vi "LaserReadContinuous.vi"() -> ()   [LabVIEW 2018]
uses:
  <vilib>/myRIO/Instrument Drivers/Onboard IO/I2C/typedefs/I2C User Configuration.ctl
  <vilib>/myRIO/Instrument Drivers/Onboard IO/I2C/typedefs/I2C Transfer Rate.ctl
  <vilib>/myRIO/Instrument Drivers/Onboard IO/I2C/typedefs/I2C Reference.ctl
  <vilib>/myRIO/Common/Instrument Driver Framework/Utilities/typedefs/myRIO Generic Hardware Reference.ctl
  <vilib>/myRIO/Common/Instrument Driver Framework/Utilities/typedefs/Hardware Version Enum.ctl
  <vilib>/myRIO/Common/Instrument Driver Framework/Utilities/typedefs/myRIO v1.0 Reference.ctl
  <vilib>/myRIO/Common/Instrument Driver Framework/Utilities/typedefs/Generic FPGA Reference.ctl
  <vilib>/myRIO/Common/Instrument Driver Framework/myRIO v1.0/I2C/typedefs/I2C Channels Enum.ctl
  <vilib>/myRIO/Instrument Drivers/Onboard IO/I2C/typedefs/I2C Configuration.ctl
  <vilib>/userdefined/High Color/nirio_resource_hc.ctl
  <vilib>/myRIO/Common/Instrument Driver Framework/myRIO v1.0/I2C/vis/myRIO v1.1 Open I2C.vi
  <vilib>/myRIO/Common/Instrument Driver Framework/Utilities/vis/Validate Channels.vi
  <vilib>/myRIO/Common/Instrument Driver Framework/myRIO v1.0/I2C/vis/myRIO v1.0 Reserve I2C.vi
  <vilib>/myRIO/Common/Instrument Driver Framework/myRIO v1.0/I2C/vis/myRIO v1.0 Close I2C.vi
  <vilib>/myRIO/Common/Instrument Driver Framework/myRIO v1.0/I2C/vis/myRIO v1.0 Build MUX Configuration I2C.vi
  <vilib>/myRIO/Common/Instrument Driver Framework/myRIO v1.0/Resource Manager/vis/myRIO v1.0 Reserve Channel List.vi
  <vilib>/myRIO/Common/Instrument Driver Framework/myRIO v1.0/I2C/vis/myRIO v1.0 Unreserve I2C.vi
  <vilib>/myRIO/Common/Instrument Driver Framework/myRIO v1.0/Resource Manager/vis/myRIO v1.0 Create Configuration List.vi
  <vilib>/myRIO/Common/Instrument Driver Framework/myRIO v1.0/Resource Manager/vis/myRIO v1.0 Reserve Channel.vi
  <vilib>/myRIO/Common/Instrument Driver Framework/myRIO v1.0/Resource Manager/vis/myRIO v1.0 Unreserve Channel.vi
  <vilib>/myRIO/Common/Instrument Driver Framework/myRIO v1.0/Resource Manager/vis/myRIO v1.0 Unreserve Channel List.vi
  <vilib>/myRIO/Common/Instrument Driver Framework/myRIO v1.0/Resource Manager/vis/myRIO v1.0 Build Mutex Name.vi
  <vilib>/Utility/VariantDataType/GetNumericInfo.vi
  <vilib>/Utility/error.llb/Error Cluster From Error Code.vi
  <vilib>/myRIO/Common/Instrument Driver Framework/myRIO v1.0/myRIO v1.1 Open.vi
  <vilib>/myRIO/Common/Instrument Driver Framework/Utilities/vis/IO Manager.vi
  <vilib>/myRIO/Common/Instrument Driver Framework/Utilities/vis/Configuration Manager.vi
  <vilib>/myRIO/Common/Instrument Driver Framework/myRIO v1.0/Resource Manager/vis/myRIO v1.0 Configure IO.vi
  <vilib>/myRIO/Common/Instrument Driver Framework/myRIO v1.0/myRIO v1.0 Close.vi
  <vilib>/myRIO/Common/Instrument Driver Framework/myRIO v1.0/I2C/vis/myRIO v1.0 Configure I2C.vi
  <vilib>/myRIO/Common/Instrument Driver Framework/myRIO v1.0/I2C/vis/myRIO v1.0 Shutdown I2C.vi
  <vilib>/myRIO/Instrument Drivers/Onboard IO/I2C/vis/myRIO I2C Open.xnode
  <vilib>/myRIO/Instrument Drivers/Onboard IO/I2C/I2C.lvlib
panel:
  out "dt":u32
  out "Waveform Chart":u16(graph)
  out "error out":errorcluster
  out "init status":bool
  out "Range":u16
  out "did_timeout":bool
  in  "stop":bool
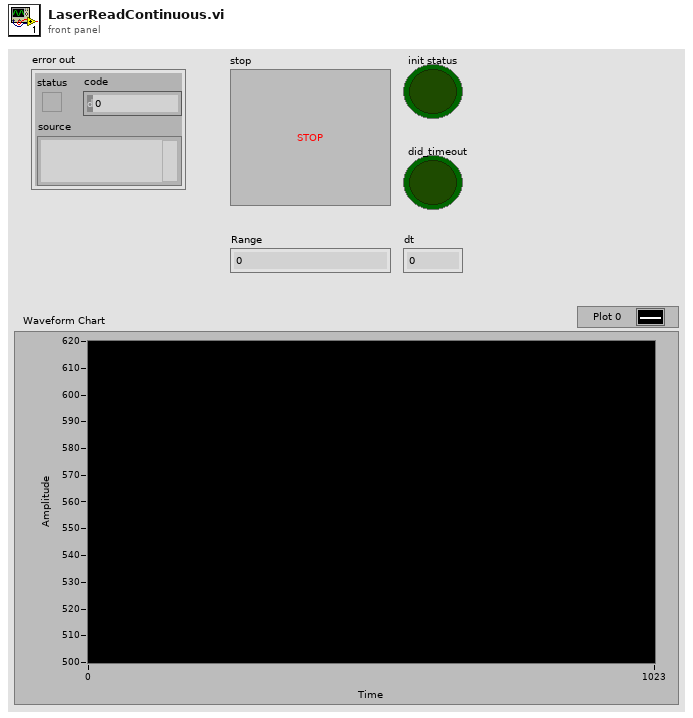
[diagram p1: front panel]
types:
  T1 = typedef "I2C.lvlib/I2C User Configuration.ctl" = cluster{"I2C Transfer Rate":T2}
  T2 = typedef "I2C.lvlib/I2C Transfer Rate.ctl" = enum16{"Standard mode (100 kbps)", "Fast mode (400 kbps)"}
  T3 = typedef "I2C.lvlib/I2C Reference.ctl" = cluster{"myRIO Reference":T4, "I2C Channels Enum":T8, "I2C Configuration":T9}
  T4 = typedef "myRIO Generic Hardware Reference.ctl" = cluster{"myRIO Model":T5, "myRIO Hardware Reference":T6}
  T5 = typedef "Hardware Version Enum.ctl" = enum16{"Unknown", "myRIO-1900", "myRIO-1950", "roboRIO", "NI ELVIS RIO CM", "ELVIS III"}
  T6 = typedef "myRIO v1.0 Reference.ctl" = cluster{"Generic FPGA Reference":T7, "Allow multiple opens":bool}
  T7 = typedef "Generic FPGA Reference.ctl" = refnum<k20>
  T8 = typedef "I2C Channels Enum.ctl" = enum16{"Not Connected", "A/I2C", "B/I2C", "I2C/I2C"}
  T9 = typedef "I2C.lvlib/I2C Configuration.ctl" = cluster{"I2C Transfer Rate":T2}
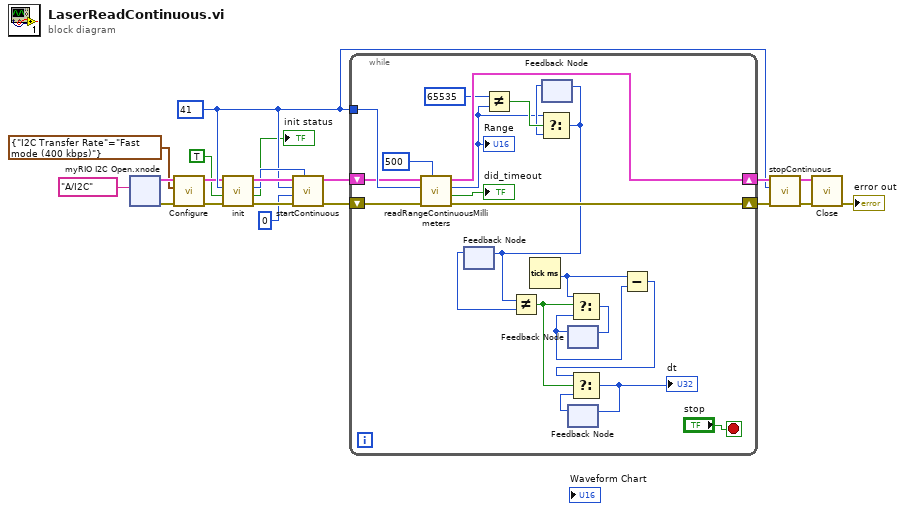
[diagram p0: block diagram]
diagram:
  w6 = u8 41
  n1 = xnode "myRIO I2C Open.xnode"("Channel Name"=tag "A/I2C") -> ("error out"=w19:errorcluster, "I2C Ref Out"=w20:T3)  [unwired: 2 in]
  n2 = call <vilib>:"Configure.vi"("error in (no error)"=w19, "I2C User Configuration"=T1 {"I2C Transfer Rate"=enum."Fast mode (400 kbps)"}, "I2C Ref In"=w20) -> ("error out"=w4:errorcluster, "I2C Ref Out"=w5:T3)  [unwired: 7 in]
  n3 = call "init.vi"("error in"=w4, "io_2V8"=TRUE, "Slave Address(7 bit)"=w6, "I2C Ref In"=w5) -> ("error out"=w9:errorcluster, "status"=→"init status":bool, "stop_variable"=w7:u8, "I2C Ref Out"=w8:T3)  [unwired: 4 in]
  n4 = call "startContinuous.vi"("stop_variable"=w7, "error in"=w9, "period_ms"=u32 0, "Slave Address(7 bit)"=w6, "I2C Ref In"=w8) -> ("error out"=w10:errorcluster, "I2C Ref Out"=w11:T3)  [unwired: 5 in]
  n5 = while {
    shift-right: [w41] -> w14
    shift-left: w11 -> [w38]
    shift-right: [w40] -> w13
    shift-left: w10 -> [w37]
    tunnel: w6 -> [w39]
    stop <- "stop" stop-if-true
    n6 = call "readRangeContinuousMillimeters.vi"("io_timeout"=u16 500 ("period_ms"), "error in"=w37, "Slave Address(7 bit)"=w39, "I2C Ref In"=w38) -> ("error out"=w40:errorcluster, "did_timeout"=→"did_timeout":bool, "Range"=w21:u16, "I2C Ref Out"=w41:T3)  [unwired: 4 in]
    "Range" <- w21
    n7 = feedback #1() -> (w31:u16)  [unwired: 1 in]
    n8 = Not Equal?(x=u16 65535 ("y"), y=w21) -> (x != y?=w33:bool)
    n9 = Tick Count (ms)() -> (millisecond timer value=w29:u32)
    n10 = feedback #2() -> (w32:u16)  [unwired: 1 in]
    n11 = Select(t=w21, s=w33, f=w32) -> (s? t:f=w23:u16)
    n12 = feedback-in #1(w23) -> ()
    n13 = Not Equal?(x=w23, y=w31) -> (x != y?=w27:bool)
    n14 = feedback-in #2(w23) -> ()
    n15 = feedback #3() -> (w28:u32)  [unwired: 1 in]
    n16 = feedback #4() -> (w26:u32)  [unwired: 1 in]
    n17 = Select(t=w29, s=w27, f=w28) -> (s? t:f=w30:u32)
    n18 = feedback-in #3(w30) -> ()
    n19 = Subtract(x=w29, y=w28) -> (x-y=w25:u32)
    n20 = Select(t=w25, s=w27, f=w26) -> (s? t:f=w24:u32)
    "dt" <- w24
    n21 = feedback-in #4(w24) -> ()
  }
  n22 = call "stopContinuous.vi"("error in"=w13, "Slave Address(7 bit)"=w6, "I2C Ref In"=w14) -> ("error out"=w15:errorcluster, "I2C Ref Out"=w16:T3)  [unwired: 7 in]
  n23 = call <vilib>:"Close.vi"("error in (no error)"=w15, "I2C Ref In"=w16) -> ("error out"=→"error out":errorcluster)  [unwired: 9 in]
